vi "_CSMObj-Add Internal Registry Rule.vi"(8 "Error In":errorcluster caption="error in (no error)", 10 "Rule":string, 11 "CSMQ In":T1={"info"={"Module Name"="", "Requested Name"="", "Group Name"="", "Mode"=enum."Stand Alone", "Allowed Messages"=[]}, "Refs"={"WatchDogQ"=refnum, "CSMDataDVR"=refnum, "Queue"={"HPriorityQ"=refnum, "LowPriorityQ"=refnum}, "GroupDataDVR"=refnum, "TagMap"=refnum, "ExitEvent"=refnum, "NewStateEvent"=refnum, "StatusChangeEvent"=refnum}}) -> (0 "error out":errorcluster, 3 "CSMQ Out":T1={"info"={"Module Name"="", "Requested Name"="", "Group Name"="", "Mode"=enum."Stand Alone", "Allowed Messages"=[]}, "Refs"={"WatchDogQ"=refnum, "CSMDataDVR"=refnum, "Queue"={"HPriorityQ"=refnum, "LowPriorityQ"=refnum}, "GroupDataDVR"=refnum, "TagMap"=refnum, "ExitEvent"=refnum, "NewStateEvent"=refnum, "StatusChangeEvent"=refnum}})   [LabVIEW 2017, in "Communicable State Machine.lvlib"]
uses:
  Communicable State Machine.lvlib
  _CSMObj.ctl
  _CSMObj-Info.ctl
  Typedef/_CSM_MODE.ctl
  _CSMObj-Refs.ctl
  _CSMObj-Data.ctl
  Priority Queue/Priority Queue.ctl
  Typedef/_Cross CSM State Data.ctl
  Typedef/_CSM_MSG_TYPE.ctl
  Typedef/_Cross CSM State Response.ctl
  Typedef/_CSM_Response Source Message.ctl
  Priority Queue/def-Data(LowPRI-Q).ctl
  _CSMObj-ModeData.ctl
  Typedef/_CSM Status Change Event Data.ctl
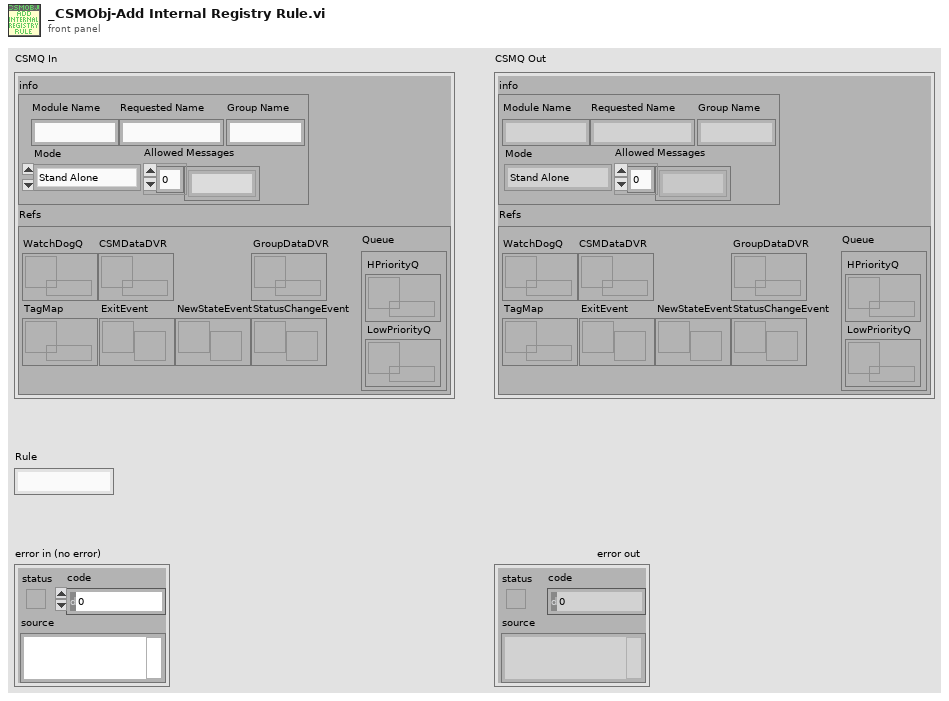
[diagram p1: front panel]
types:
  T1 = typedef "Communicable State Machine.lvlib/_CSMObj.ctl" = cluster{"info":T2, "Refs":T4}
  T2 = typedef "Communicable State Machine.lvlib/_CSMObj-Info.ctl" = cluster{"Module Name":string, "Requested Name":string, "Group Name":string, "Mode":T3, "Allowed Messages":string[]}
  T3 = typedef "Communicable State Machine.lvlib/_CSM_MODE.ctl" = enum16{"Not Exist", "Stand Alone", "CSM", "Worker", "Worker Agent", "Chain Node", "Chain"}
  T4 = typedef "Communicable State Machine.lvlib/_CSMObj-Refs.ctl" = cluster{"WatchDogQ":refnum<queue>, "CSMDataDVR":refnum<data-value>, "Queue":T5, "GroupDataDVR":refnum<data-value>, "TagMap":refnum<data-value>, "ExitEvent":refnum<user-event>, "NewStateEvent":refnum<user-event>, "StatusChangeEvent":refnum<user-event>}
  T5 = typedef "Communicable State Machine.lvlib/Priority Queue.ctl" = cluster{"HPriorityQ":refnum<queue>, "LowPriorityQ":refnum<queue>}
  T6 = typedef "Communicable State Machine.lvlib/_CSMObj-Data.ctl" = cluster{"RemoteMessge?":bool, "error":errorcluster, "InternalRegistryRules":string[], "Return State":string, "Initialized":enum16{"Initializing", "Ready", "Exiting"}}
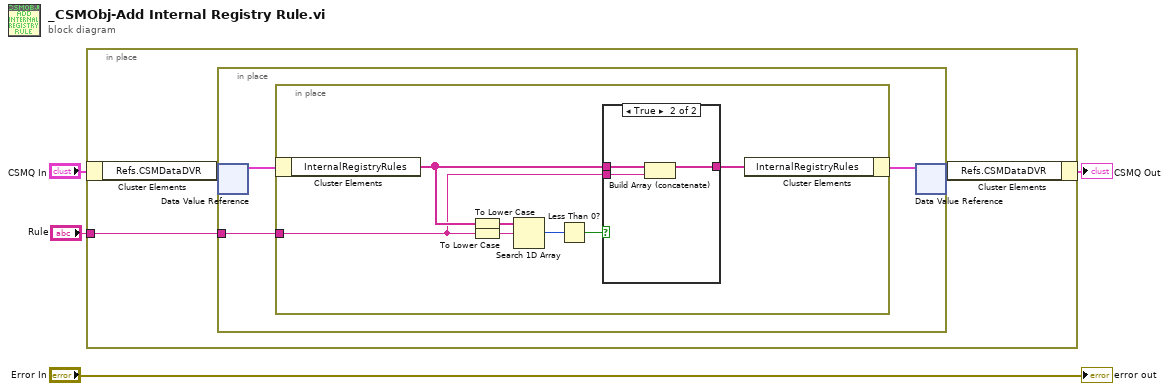
[diagram p0: block diagram]
diagram:
  n1 = in-place "In Place Element Structure" {
    in-place-border: "Rule" -> [w5]
    n2 = in-place-cluster #1("CSMQ In") -> ("Refs.CSMDataDVR"=w7:refnum<data-value>)
    n3 = in-place {
      in-place-border: w5 -> [w8]
      n4 = in-place-dvr #2(w7) -> (w10:T6)  [unwired: 1 out]
      n5 = in-place {
        in-place-border: w8 -> [w13]
        n6 = in-place-cluster #3(w10) -> ("InternalRegistryRules"=w15:string[])
        n7 = To Lower Case(string=w15) -> (all lower case string=w17:string[])
        n8 = To Lower Case(string=w13) -> (all lower case string=w16:string)
        n9 = Search 1D Array(1D array=w17, element=w16) -> (index of element=w12:i32)  [unwired: 1 in]
        n10 = Less Than 0?(x=w12) -> (x < 0?=w11:bool)
        n11 = case shown="True" w11 {
          tunnel: w15 -> [w18 w21]
          tunnel: [w18 w20] -> w14
          tunnel: w13 -> [_ w19]
          frame False {
          }
          frame True {
            n12 = Build Array (concatenate)(w21, w19) -> (w20:string[])
          }
        }
        n13 = in-place-cluster #3("InternalRegistryRules"=w14) -> (w9:T6)
      }
      n14 = in-place-dvr #2(w9) -> (w6:refnum<data-value>)  [unwired: 1 out]
    }
    n15 = in-place-cluster #1("Refs.CSMDataDVR"=w6) -> (→"CSMQ Out":T1)
  }
  "error out" <- "Error In"
